vi "Periodic Tasks.vi"(8 "error in":errorcluster) -> ()   [LabVIEW 2014]
doc: "This VI runs in parallel to other tasks. It can contain as many user-defined periodic loops as you need. These can carry out PID or other sorts of timed response."
uses:
  LED_Colors.ctl
  LED_Patterns.ctl
  LED Message.ctl
  <vilib>/NI/AMC/Create Single Message.vi
  <vilib>/NI/AMC/Update Message Routing Info.vi
  <vilib>/NI/AMC/Read Termination Message.vi
  <vilib>/Rock Robotics/WPI/Joystick/WPI_JoystickGetSetRefNum.vi
  <vilib>/Rock Robotics/WPI/RobotDrive/WPI_RobotDriveGetSetRefNum.vi
  <vilib>/NI/AMC/Send Message.vi
  <vilib>/NI/AMC/Globals.vi
  <vilib>/NI/AMC/AMC.lvlib
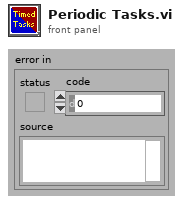
[diagram p1: front panel]
types:
  T1 = typedef "WPI_JoystickDevRef.ctl" = cluster{"Device":T2}
  T2 = typedef "WPI_JoystickDeviceEnum.ctl" = enum16{"USB 0", "USB 1", "USB 2", "USB 3", "USB 4", "USB 5"}
  T3 = typedef "WPI_RobotDriveDevRef.ctl" = cluster{"DevStatus":errorcluster, "Motors[]":T4[], "Square Inputs":bool, "Max Output":dbl}
  T4 = typedef "WPI_MotorControlDeviceRef.ctl" = cluster{"DeviceStatus":errorcluster, "Type":T5, "PWM":cluster{"Controller":T6, "PWM Channel":T7, "DeadBand":T8}, "CAN":cluster{"Device Number":u8, "Control Mode":T9, "Semaphore":T10, "Max Vout":dbl, "TalonSRX Control Mode":T11}, "Invert":bool, "TransformRef":T12, "InvTransformRef":T12}
  T5 = typedef "WPI_MotorControlType.ctl" = enum16{"PWM", "CAN", "CANTalonSRX"}
  T6 = typedef "FPGA_TypedefDigitalModule.ctl" = enum16{"Controller 1"}
  T7 = typedef "FPGA_DIOPWMChannel.ctl" = enum8{"PWM 0", "PWM 1", "PWM 2", "PWM 3", "PWM 4", "PWM 5", "PWM 6", "PWM 7", "PWM 8", "PWM 9", "PWM MXP 0", "PWM MXP 1", "PWM MXP 2", "PWM MXP 3", "PWM MXP 4", "PWM MXP 5", "PWM MXP 6", "PWM MXP 7", "PWM MXP 8", "PWM MXP 9", "Invalid"}
  T8 = typedef "WPI_PWMDeadband.ctl" = cluster{"Name":string, "maxPositivePwm":i32, "minPositivePwm":i32, "centerPwm":i32, "maxNegativePwm":i32, "minNegativePwm":i32, "angularRange":u16}
  T9 = typedef "WPI_CANJaguar_ControlMode.ctl" = enum8{"Percent VBus", "Current", "Speed", "Position", "Voltage"}
  T10 = typedef "Semaphore RefNum" = refnum<k1>
  T11 = typedef "WPI_CANTalonSRX_APIControlMode.ctl" = enum8{"Percent VBus", "Speed", "Position", "Slave", "Unchanged / Invalid"}
  T12 = typedef "WPI_PWMTransform_ConPane.ctl" = refnum<vi>
  T13 = typedef "AMC.lvlib/Message Queue.ctl" = refnum<queue>
  T14 = cluster{"JoystickDevRef":T1, "RobotDriveDevRef":T3}
  T15 = typedef "WPI_DriverStationRobotMode2.ctl" = enum16{"Autonomous Disabled", "Autonomous Enabled", "Teleop Disabled", "Teleop Enabled", "Disconnected", "Finish", "Test Disabled", "Test Enabled", "Emergency Stopped"}
  T16 = typedef "LED_Patterns.ctl" = enum8{"Black White", "Solid", "Blink", "Sweep", "Sleep"}
  T17 = typedef "LED_Colors.ctl" = enum8{"Red", "Green", "Blue", "Cyan", "Magenta", "Yellow"}
  T18 = typedef "LED Message.ctl" = cluster{"Pattern":T16, "Color":T17, "Section":u8}
  T19 = typedef "WPI_I2CDevRef.ctl" = cluster{"DevStatus":errorcluster, "Controller":T6, "Device Address":u8, "Handle":i32, "I2C Bus":T20}
  T20 = typedef "i2c_bus.ctl" = enum16{"I2C On-Board", "I2C MXP", "Invalid"}
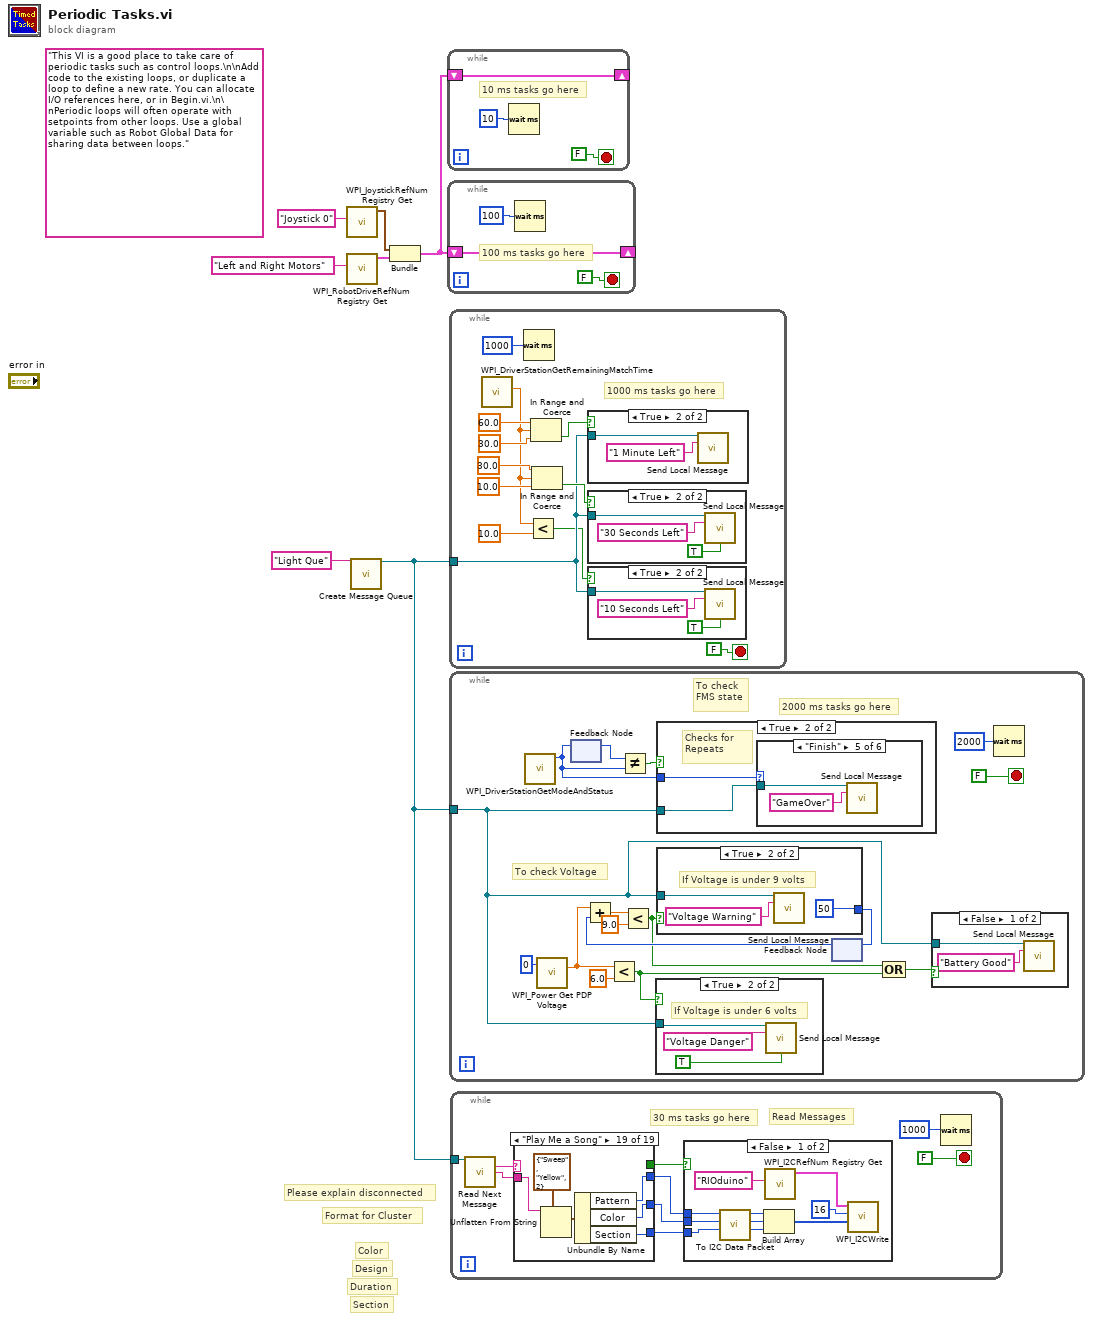
[diagram p0: block diagram]
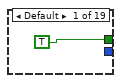
[diagram p3: hidden frame]
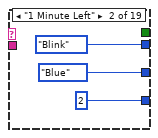
[diagram p4: hidden frame]
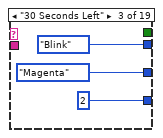
[diagram p5: hidden frame]
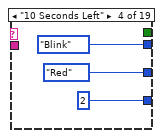
[diagram p6: hidden frame]
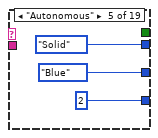
[diagram p7: hidden frame]
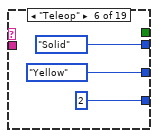
[diagram p8: hidden frame]
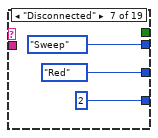
[diagram p9: hidden frame]
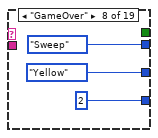
[diagram p10: hidden frame]
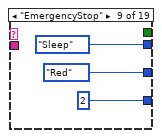
[diagram p11: hidden frame]
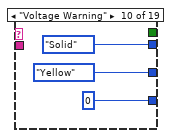
[diagram p12: hidden frame]
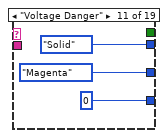
[diagram p13: hidden frame]
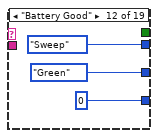
[diagram p14: hidden frame]
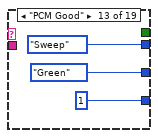
[diagram p15: hidden frame]
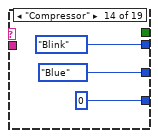
[diagram p16: hidden frame]
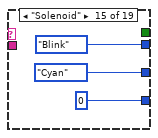
[diagram p17: hidden frame]
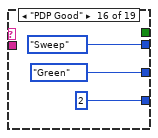
[diagram p18: hidden frame]
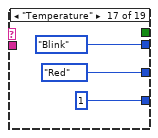
[diagram p19: hidden frame]
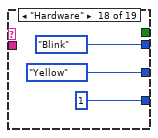
[diagram p20: hidden frame]
diagram:
  (unwired) "This VI is a good place to take care of periodic tasks such as control loops.\n\nAdd code to the existing loops, or duplicate a loop to define a new rate. You can allocate I/O references here, or in Begin.vi.\n\nPeriodic loops will often operate with setpoints from other loops. Use a global variable such as Robot Global Data for sharing data between loops."
  # "Please explain disconnected"
  # "Color"
  # "Design"
  # "Section"
  # "Format for Cluster"
  # "Duration"
  n1 = call <vilib>:"WPI_JoystickRefNum Registry Get.vi"("refnum name"="Joystick 0") -> ("JoystickDevRef"=w5:T1)  [unwired: 1 in, 9 out]
  n2 = call <vilib>:"WPI_RobotDriveRefNum Registry Get.vi"("refnum name"="Left and Right Motors") -> ("RobotDriveDevRef"=w4:T3)  [unwired: 1 in, 9 out]
  n3 = call <vilib>:"Create Message Queue.vi"("message queue name"="Light Que") -> ("message queue out"=w2:T13)  [unwired: 13 in, 1 out]
  n4 = Bundle("JoystickDevRef"=w5, "RobotDriveDevRef"=w4) -> (w3:T14)  [unwired: 1 out]
  n5 = while {
    shift-right: [w8] -> _
    shift-left: w3 -> [w8]
    stop <- FALSE stop-if-true
    # "10 ms tasks go here"
    n6 = Wait (ms)(milliseconds to wait=u32 10) -> ()  [unwired: 1 out]
  }
  n7 = while {
    shift-right: [w11] -> _
    shift-left: w3 -> [w11]
    stop <- FALSE stop-if-true
    # "100 ms tasks go here"
    n8 = Wait (ms)(milliseconds to wait=u32 100) -> ()  [unwired: 1 out]
  }
  n9 = while {
    tunnel: w2 -> [w17]
    stop <- FALSE stop-if-true
    # "1000 ms tasks go here"
    n10 = call <vilib>:"WPI_DriverStationGetRemainingMatchTime.vi"() -> ("Match Time(s)"=w15:sgl)  [unwired: 10 in, 1 out]
    n11 = Wait (ms)(milliseconds to wait=u32 1000) -> ()  [unwired: 1 out]
    n12 = Less?(x=w15, y=sgl 10.0) -> (x < y?=w14:bool)
    n13 = In Range and Coerce(upper limit=sgl 60.0 ("y"), x=w15, lower limit=sgl 30.0 ("y")) -> (In Range?=w21:bool)  [unwired: 1 out]
    n14 = In Range and Coerce(upper limit=sgl 30.0 ("y"), x=w15, lower limit=sgl 10.0 ("y")) -> (In Range?=w18:bool)  [unwired: 1 out]
    n15 = case shown="True" w21 {
      tunnel: w17 -> [_ w33]
      frame False {
      }
      frame True {
        n16 = call <vilib>:"Send Local Message.vi"("message queue in"=w33, "message name"="1 Minute Left") -> ()  [unwired: 11 in, 3 out]
      }
    }
    n17 = case shown="True" w18 {
      tunnel: w17 -> [_ w31]
      frame False {
      }
      frame True {
        n18 = call <vilib>:"Send Local Message.vi"("message queue in"=w31, "message name"="30 Seconds Left", "priority message (F)"=TRUE) -> ()  [unwired: 10 in, 3 out]
      }
    }
    n19 = case shown="True" w14 {
      tunnel: w17 -> [_ w28]
      frame False {
      }
      frame True {
        n20 = call <vilib>:"Send Local Message.vi"("message queue in"=w28, "message name"="10 Seconds Left", "priority message (F)"=TRUE) -> ()  [unwired: 10 in, 3 out]
      }
    }
  }
  n21 = while {
    tunnel: w2 -> [w36]
    stop <- FALSE stop-if-true
    # "2000 ms tasks go here"
    # "To check \nFMS state"
    # "To check Voltage"
    n22 = call <vilib>:"WPI_DriverStationGetModeAndStatus.vi"() -> ("Robot Mode"=w39:T15)  [unwired: 10 in, 1 out]
    n23 = call <vilib>:"WPI_Power Get PDP Voltage.vi"("Power Distribution Panel (0)"=u8 0) -> ("voltage (V)"=w46:dbl)  [unwired: 13 in, 1 out]
    n24 = feedback-in #1(w39) -> ()
    n25 = feedback #1() -> (w38:T15)  [unwired: 1 in]
    n26 = Less?(x=w46, y=6.0) -> (x < y?=w34:bool)
    n27 = Not Equal?(x=w38, y=w39) -> (x != y?=w40:bool)
    n28 = case shown="True" w34 {
      tunnel: w36 -> [_ w66]
      frame False {
      }
      frame True {
        # "If Voltage is under 6 volts"
        n29 = call <vilib>:"Send Local Message.vi"("message queue in"=w66, "message name"="Voltage Danger", "priority message (F)"=TRUE) -> ()  [unwired: 10 in, 3 out]
      }
    }
    n30 = case shown="True" w40 {
      tunnel: w39 -> [_ w52]
      tunnel: w36 -> [_ w53]
      frame False {
        # "Its a repeat"
      }
      frame True {
        # "Checks for\nRepeats"
        n31 = case shown="\"Finish\"" w52 {
          tunnel: w53 -> [_ w55 w57 w59 w61 w63]
          frame Default {
          }
          frame "Autonomous Enabled" {
            n32 = call <vilib>:"Send Local Message.vi"("message queue in"=w55, "message name"="Autonomous") -> ()  [unwired: 11 in, 3 out]
          }
          frame "Teleop Enabled" {
            n33 = call <vilib>:"Send Local Message.vi"("message queue in"=w57, "message name"="Teleop") -> ()  [unwired: 11 in, 3 out]
          }
          frame "Disconnected" {
            n34 = call <vilib>:"Send Local Message.vi"("message queue in"=w59, "message name"="Disconnected") -> ()  [unwired: 11 in, 3 out]
          }
          frame "Finish" {
            n35 = call <vilib>:"Send Local Message.vi"("message queue in"=w61, "message name"="GameOver") -> ()  [unwired: 11 in, 3 out]
          }
          frame "Emergency Stopped" {
            n36 = call <vilib>:"Send Local Message.vi"("message queue in"=w63, "message name"="EmergencyStop") -> ()  [unwired: 11 in, 3 out]
          }
        }
      }
    }
    n37 = feedback #2() -> (w48:i32)  [unwired: 1 in]
    n38 = Add(x=w46, y=w48) -> (x+y=w47:dbl)
    n39 = Less?(x=w47, y=9.0) -> (x < y?=w35:bool)
    n40 = case shown="True" w35 {
      tunnel: w36 -> [_ w70]
      tunnel: [0 50] -> w49
      frame False {
      }
      frame True {
        # "If Voltage is under 9 volts"
        n41 = call <vilib>:"Send Local Message.vi"("message queue in"=w70, "message name"="Voltage Warning") -> ()  [unwired: 11 in, 3 out]
      }
    }
    n42 = feedback-in #2(w49) -> ()
    n43 = Compound Arithmetic op=OR(w35, w34) -> (w37:bool)
    n44 = case shown="False" w37 {
      tunnel: w36 -> [w50 _]
      frame False {
        n45 = call <vilib>:"Send Local Message.vi"("message queue in"=w50, "message name"="Battery Good") -> ()  [unwired: 11 in, 3 out]
      }
      frame True {
      }
    }
    n46 = Wait (ms)(milliseconds to wait=u32 2000) -> ()  [unwired: 1 out]
  }
  n47 = while {
    tunnel: w2 -> [w79]
    stop <- FALSE stop-if-true
    # "Read Messages"
    # "30 ms tasks go here"
    n48 = call <vilib>:"Read Next Message.vi"("message queue in"=w79) -> ("message name"=w78:string, "message value"=w71:string)  [unwired: 7 in, 6 out]
    n49 = case shown="\"Play Me a Song\"" w78 {
      tunnel: [_ LED_Patterns."Blink" ("Pattern 2") LED_Patterns."Blink" ("Pattern 3") LED_Patterns."Blink" ("Pattern 3") LED_Patterns."Solid" ("Pattern 4") LED_Patterns."Solid" ("Pattern 5") LED_Patterns."Sweep" ("Pattern 6") LED_Patterns."Sweep" ("Pattern 7") LED_Patterns."Sleep" ("Pattern 8") LED_Patterns."Solid" ("Pattern 9") LED_Patterns."Solid" ("Pattern 10") LED_Patterns."Sweep" ("Pattern 10") LED_Patterns."Sweep" ("Pattern 10") LED_Patterns."Blink" ("Pattern") LED_Patterns."Blink" ("Pattern") LED_Patterns."Sweep" ("Pattern") LED_Patterns."Blink" ("Pattern") LED_Patterns."Blink" ("Pattern") w142] -> w75
      tunnel: [_ LED_Colors."Blue" ("1 Minute Left") LED_Colors."Magenta" ("30 Sec left") LED_Colors."Red" ("30 Sec left") LED_Colors."Blue" ("Auto") LED_Colors."Yellow" ("Teleop") LED_Colors."Red" ("Disconnected") LED_Colors."Yellow" ("GAME OVER") LED_Colors."Red" ("Critical ERROR") LED_Colors."Yellow" ("Battery Warning") LED_Colors."Magenta" ("Low Battery") LED_Colors."Green" ("Low Battery") LED_Colors."Green" ("Low Battery") LED_Colors."Blue" ("Hardware") LED_Colors."Cyan" ("Hardware") LED_Colors."Green" ("Hardware") LED_Colors."Red" ("Hardware") LED_Colors."Yellow" ("Hardware") w144] -> w74
      tunnel: [_ u8 2 ("Section 2") u8 2 ("Section 3") u8 2 ("Section 3") u8 2 ("Section 4") u8 2 ("Section 5") u8 2 ("Section 6") u8 2 ("Section 7") u8 2 ("Section 8") u8 0 ("Section 9") u8 0 ("Section 10") u8 0 ("Section 10") u8 1 ("Section 10") u8 0 ("Section") u8 0 ("Section") u8 2 ("Section") u8 1 ("Section") u8 1 ("Section") w143] -> w73
      tunnel: [TRUE _ _ _ _ _ _ _ _ _ _ _ _ _ _ _ _ _ _] -> w72
      tunnel: w71 -> [_ _ _ _ _ _ _ _ _ _ _ _ _ _ _ _ _ _ w147]
      frame Default {
      }
      frame "1 Minute Left" {
      }
      frame "30 Seconds Left" {
      }
      frame "10 Seconds Left" {
      }
      frame "Autonomous" {
      }
      frame "Teleop" {
      }
      frame "Disconnected" {
      }
      frame "GameOver" {
      }
      frame "EmergencyStop" {
      }
      frame "Voltage Warning" {
      }
      frame "Voltage Danger" {
      }
      frame "Battery Good" {
      }
      frame "PCM Good" {
      }
      frame "Compressor" {
      }
      frame "Solenoid" {
      }
      frame "PDP Good" {
      }
      frame "Temperature" {
      }
      frame "Hardware" {
      }
      frame "Play Me a Song" {
        n50 = Unflatten From String(type=T18 {"Pattern"=enum."Sweep", "Color"=enum."Yellow", "Section"=2} ("LED Message"), binary string=w147) -> (value=w145:T18)  [unwired: 3 in, 2 out]
        n51 = Unbundle By Name(w145) -> ("Pattern"=w142:T16, "Color"=w144:T17, "Section"=w143:u8)
      }
    }
    n52 = case shown="False" w72 {
      tunnel: w75 -> [w81 _]
      tunnel: w74 -> [w80 _]
      tunnel: w73 -> [w82 _]
      frame False {
        n53 = call "To I2C Data Packet.vi"("Section"=w82, "Color"=w80, "Pattern"=w81) -> ("Output Byte 3"=w87:u8, "Output Byte 2"=w88:u8, "Output Byte"=w89:u8)  [unwired: 6 in]
        n54 = Build Array(w89, w88, w87) -> (w86:u8[])
        n55 = call <vilib>:"WPI_I2CRefNum Registry Get.vi"("refnum name"="RIOduino") -> ("I2CDevRef"=w85:T19)  [unwired: 9 in, 1 out]
        n56 = call <vilib>:"WPI_I2CWrite.vi"("I2CDataToSend"=w86, "I2CRegister"=u8 16, "I2CDevRef"=w85) -> ()  [unwired: 7 in, 2 out]
      }
      frame True {
      }
    }
    n57 = Wait (ms)(milliseconds to wait=u32 1000) -> ()  [unwired: 1 out]
  }
